vi "Set Preferred Steering Angles.vi"(8 "error in (no error)":errorcluster, 10 "preferred steering angles":dbl[](array[numeric]), 11 "steering frame in":refnum<class "NI_Robotics_Steering Frame.lvclass">) -> (0 "error out":errorcluster, 3 "steering frame out":refnum<class "NI_Robotics_Steering Frame.lvclass">)   [LabVIEW 2017, in "NI_Robotics_Steering Frame.lvclass"]
uses:
  <vilib>/robotics/Steering/Steering Frame/NI_Robotics_Steering Frame.lvclass
  <vilib>/robotics/Steering/Steering Frame/NI_Robotics_Steering Frame.lvclass/NI_Robotics_Steering Frame.ctl
  <vilib>/robotics/Steering/Wheel/NI_Robotics_Wheel.lvclass
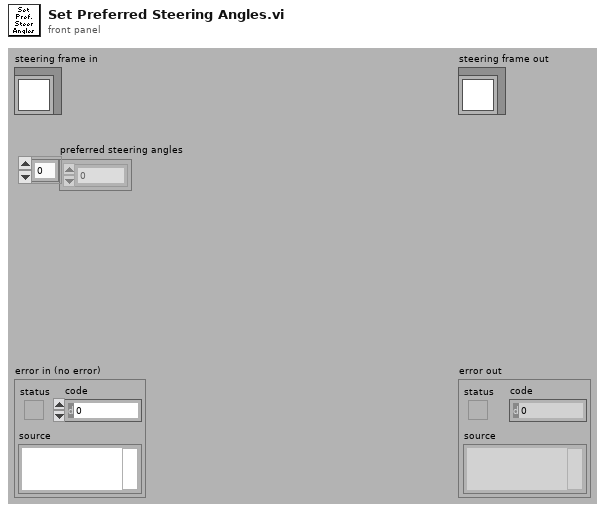
[diagram p1: front panel]
types:
  T1 = typedef "NI_Robotics_Steering Frame.lvclass/Wheel Orientation.ctl" = cluster{"wheel":refnum<class "NI_Robotics_Wheel.lvclass">, "x position":dbl, "y position":dbl, "frame angle (rad)":dbl}
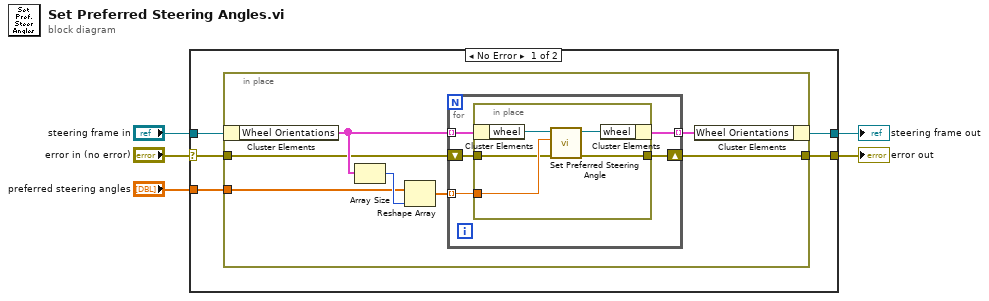
[diagram p0: block diagram]
diagram:
  n1 = case shown="No Error" "error in (no error)" {
    selector: "error in (no error)" -> [w6 w29]
    tunnel: [w7 w29] -> w4
    tunnel: [w9 w28] -> w2
    tunnel: "steering frame in" -> [w10 w28]
    tunnel: "preferred steering angles" -> [w8 _]
    frame No Error {
      n2 = in-place {
        in-place-border: w8 -> [w14]
        in-place-border: [w12] -> w7
        in-place-border: w6 -> [w11]
        n3 = in-place-cluster #1(w10) -> ("Wheel Orientations"=w16:T1[])
        n4 = Array Size(array=w16) -> (size(s)=w15:i32)
        n5 = Reshape Array(w14, w15) -> (w13:dbl[])
        n6 = for {
          tunnel: w16 -> [w22] mode=indexing
          tunnel: w13 -> [w20] mode=indexing
          tunnel: [w21] -> w17 mode=indexing
          shift-right: [w19] -> w12
          shift-left: w11 -> [w18]
          n7 = in-place {
            in-place-border: w20 -> [w25]
            in-place-border: [w24] -> w19
            in-place-border: w18 -> [w23]
            n8 = in-place-cluster #2(w22) -> ("wheel"=w27:refnum<class "NI_Robotics_Wheel.lvclass">)
            n9 = call-dynamic "Set Preferred Steering Angle.vi"("error in (no error)"=w23, "preferred steering angle (rad)"=w25, "wheel in"=w27) -> ("error out"=w24:errorcluster, "wheel out"=w26:refnum<class "NI_Robotics_Wheel.lvclass">)  [unwired: 7 in]
            n10 = in-place-cluster #2("wheel"=w26) -> (w21:T1)
          }
        }
        n11 = in-place-cluster #1("Wheel Orientations"=w17) -> (w9:refnum<class "NI_Robotics_Steering Frame.lvclass">)
      }
    }
    frame Error {
    }
  }
  "error out" <- w4
  "steering frame out" <- w2
